vi "HEWH Source String Array.vi"(0 "GEA2 HyperData":bool, 5 "Pannel List":string[](array[string])) -> (8 "Source Array":string[](array[string]))   [LabVIEW 2013]
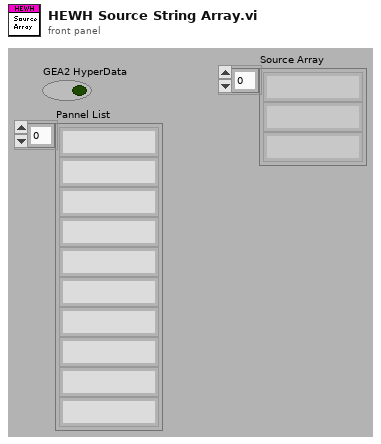
[diagram p1: front panel]
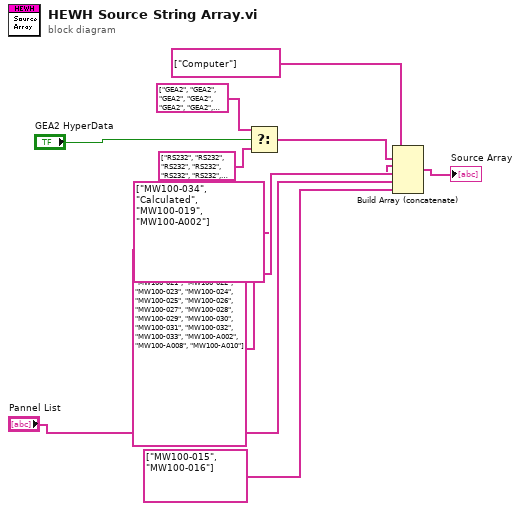
[diagram p0: block diagram]
diagram:
  n1 = Select(t=string[] ["GEA2", "GEA2", "GEA2", "GEA2", "GEA2", "GEA2", "GEA2", "GEA2", "GEA2", "GEA2", "GEA2", "GEA2", "GEA2", "GEA2", "GEA2"], s="GEA2 HyperData", f=string[] ["RS232", "RS232", "RS232", "RS232", "RS232", "RS232", "RS232", "RS232", "RS232", "RS232", "RS232", "RS232"]) -> (s? t:f=w6:string[])
  n2 = Build Array (concatenate)(string[] ["Computer"] ("array"), w6, string[] ["MW100-034", "Calculated", "MW100-019", "MW100-A002"], string[] ["MW100-011", "MW100-012", "MW100-013", "MW100-015", "MW100-016", "MW100-017", "MW100-021", "MW100-022", "MW100-023", "MW100-024", "MW100-025", "MW100-026", "MW100-027", "MW100-028", "MW100-029", "MW100-030", "MW100-031", "MW100-032", "MW100-033", "MW100-A002", "MW100-A008", "MW100-A010"] ("Array"), "Pannel List", string[] ["MW100-015", "MW100-016"] ("Array")) -> (→"Source Array":string[])
